vi "FTW-EventLogger-Shutdown.vi"(0 "Event Logger API":refnum<class "FTW-EventLogger-API.lvclass">, 11 "error in":errorcluster) -> (4 "Event Logger API out":refnum<class "FTW-EventLogger-API.lvclass">, 15 "error out":errorcluster)   [LabVIEW 2013, in "FTW-EventLogger-API.lvclass"]
doc: "This method destroys the Logger Process that is referred to by the input LoggerID. This method should be called as one of the very last tasks in your application. Until this method is called, the Logger Process will maintain an open file handle to the logfile; once this method has been called, the file handle is released."
uses:
  FTW-EventLogger-API.lvclass
  FTW-EventLogger-API.lvclass/FTW-EventLogger-API.ctl
  Messaging/Messenger.Actor/FTW-Messenger-Actor.lvclass
panel:
  # "Inputs"
  # "Outputs"
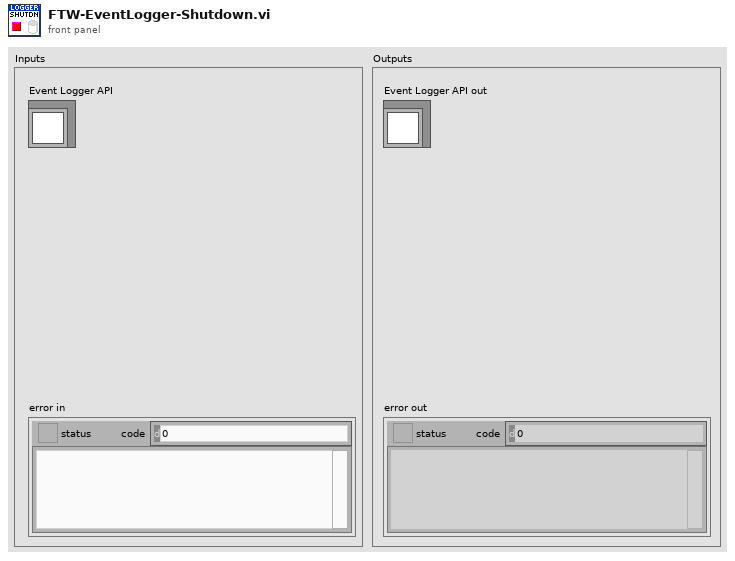
[diagram p1: front panel]
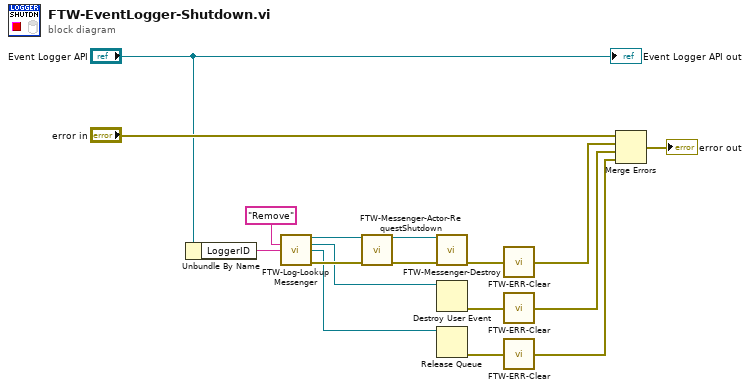
[diagram p0: block diagram]
diagram:
  n1 = Unbundle By Name("Event Logger API") -> ("LoggerID"=w1:string)
  n2 = call "FTW-Log-LookupMessenger.vi"("Action"="Remove", "LoggerID"=w1) -> ("Logger Messenger out"=w15:refnum<class "FTW-Messenger-Actor.lvclass">, "Logged Event Broadcast"=w10:refnum<user-event>, "Log Queue"=w9:refnum<queue>, "error out"=w13:errorcluster)  [unwired: 10 in]
  n3 = call-dynamic "FTW-Messenger-Actor-RequestShutdown.vi"("Messenger"=w15, "error in"=w13) -> ("Messenger out"=w14:refnum<class "FTW-Messenger-Actor.lvclass">, "error out"=w12:errorcluster)  [unwired: 12 in]
  n4 = call-dynamic "FTW-Messenger-Destroy.vi"("Messenger"=w14, "error in"=w12) -> ("error out"=w8:errorcluster)  [unwired: 13 in]
  n5 = Destroy User Event(user event=w10) -> (error out=w6:errorcluster)  [unwired: 1 in]
  n6 = Release Queue(queue=w9) -> (error out=w5:errorcluster)  [unwired: 2 in, 2 out]
  n7 = call "FTW-ERR-Clear.vi"("error to snuff"=w8) -> ("no error"=w7:errorcluster)
  n8 = call "FTW-ERR-Clear.vi"("error to snuff"=w6) -> ("no error"=w3:errorcluster)
  n9 = call "FTW-ERR-Clear.vi"("error to snuff"=w5) -> ("no error"=w4:errorcluster)
  n10 = Merge Errors("error in", w7, w3, w4) -> (→"error out":errorcluster)
  "Event Logger API out" <- "Event Logger API"
